vi "FTW-Actor-Log-Job.vi"(0 "FTW Actor Instance":refnum<class "FTW-ActorInstance.lvclass">, 5 "Job Name":string, 7 "Job Data":string, 11 "error in":errorcluster) -> (4 "FTW Actor Instance out":refnum<class "FTW-ActorInstance.lvclass">, 15 "error out":errorcluster)   [LabVIEW 2015, in "FTW-ActorInstance.lvclass"]
uses:
  FTW-ActorInstance.lvclass
  FTW-ActorInstance.lvclass/FTW-ActorInstance.ctl
  FTW-Actor-FrameworkEvent.ctl
panel:
  # "Inputs"
  # "Outputs"
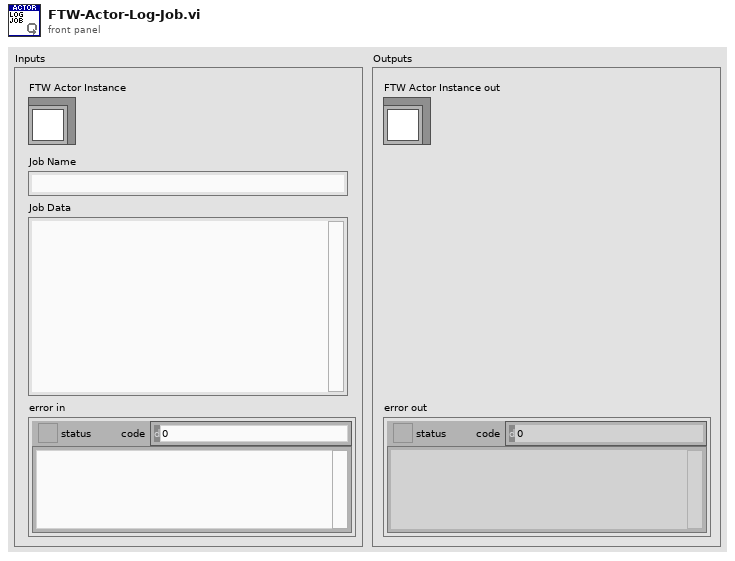
[diagram p1: front panel]
types:
  T1 = typedef "FTW-ActorInstance.lvclass/FTW-Actor-FrameworkEvent.ctl" = enum16{"Instance Initializing", "Instance Constructed", "Instance Initialized", "Instance Job", "Instance Handle Request", "Instance Shutting Down", "Instance Destroyed"}
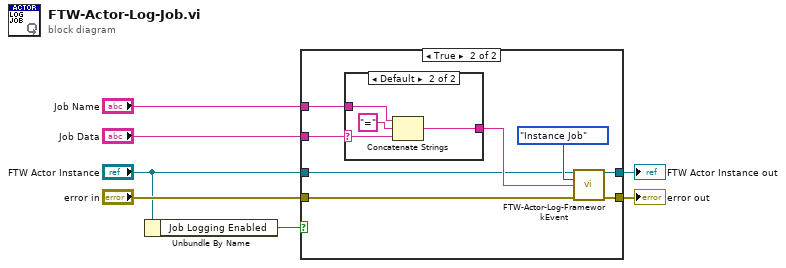
[diagram p0: block diagram]
diagram:
  n1 = Unbundle By Name("FTW Actor Instance") -> ("Job Logging Enabled"=w1:bool)
  n2 = case shown="True" w1 {
    tunnel: [w9 w17] -> w7
    tunnel: "error in" -> [w8 w16]
    tunnel: [w8 w15] -> w5
    tunnel: "Job Data" -> [_ w13]
    tunnel: "Job Name" -> [_ w12]
    tunnel: "FTW Actor Instance" -> [w9 w10]
    frame False {
    }
    frame True {
      n3 = case shown="Default" w13 {
        selector: w13 -> [_ w22]
        tunnel: w12 -> [w18 w21]
        tunnel: [w18 w19] -> w11
        frame "" {
        }
        frame Default {
          n4 = Concatenate Strings(w21, "=" ("string"), w22) -> (w19:string)
        }
      }
      n5 = call "FTW-Actor-Log-FrameworkEvent.vi"("FTW Actor Instance"=w10, "Framework Event"=FTW-Actor-FrameworkEvent."Instance Job", "Event Data"=w11, "error in"=w16) -> ("FTW Actor Instance out"=w17:refnum<class "FTW-ActorInstance.lvclass">, "error out"=w15:errorcluster)  [unwired: 10 in]
    }
  }
  "error out" <- w5
  "FTW Actor Instance out" <- w7
